vi "Read ZM_state.vi"(8 "error in (no error)":errorcluster, 11 "HE_state in":refnum<class "HE_state_v2.lvclass">) -> (0 "error out":errorcluster, 2 "HE_ZM_state":refnum<class "HE_ZM_state.lvclass">, 3 "HE_state out":refnum<class "HE_state_v2.lvclass">)   [LabVIEW 2019]
uses:
  HE_state_v2.lvclass
  C:/my_projects/projects/Algorithms/Labview/19/Heating/heating1/Z_state_v2/HE_Z_state_v2.lvclass
  C:/my_projects/projects/Algorithms/Labview/19/Heating/heating1/ZM_state/HE_ZM_state.lvclass
  C:/my_projects/projects/Algorithms/Labview/19/Sequence/State/State.lvclass
  ZM_state/HE_ZM_state.lvclass
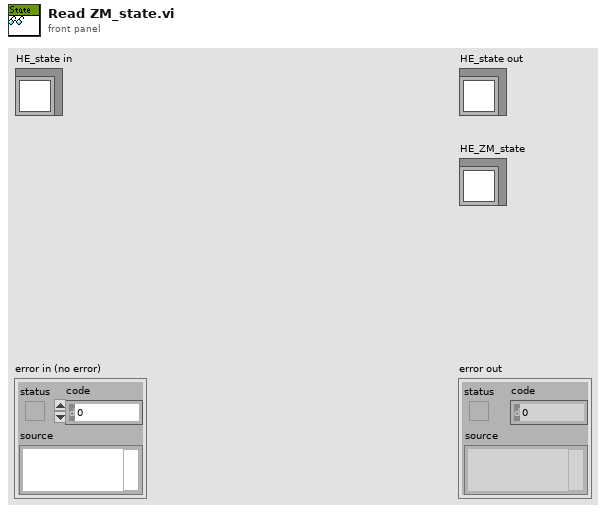
[diagram p1: front panel]
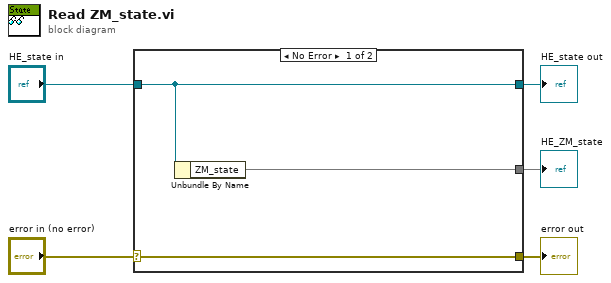
[diagram p0: block diagram]
diagram:
  n1 = case shown="No Error" "error in (no error)" {
    selector: "error in (no error)" -> [w8 w9]
    tunnel: [w8 w9] -> w4
    tunnel: [w7 w10] -> w2
    tunnel: "HE_state in" -> [w7 w10]
    tunnel: [w6 _] -> w1
    frame No Error {
      n2 = Unbundle By Name(w7) -> ("ZM_state"=w6)
    }
    frame Error {
    }
  }
  "error out" <- w4
  "HE_state out" <- w2
  "HE_ZM_state" <- w1
